vi "CDMA_RxDemodulate.vi"(8 "error in (no error)":errorcluster caption="错误输入（无错误）", 9 "pichData":cdb[](array[numeric]), 10 "dpchData":cdb[](array[numeric]), 11 "Path In":path) -> (0 "error out":errorcluster caption="错误输出", 1 "data1A":cdb[](array[numeric]), 2 "dpchBit":dbl[](array[numeric]), 3 "Path  Out":path)   [LabVIEW 2015]
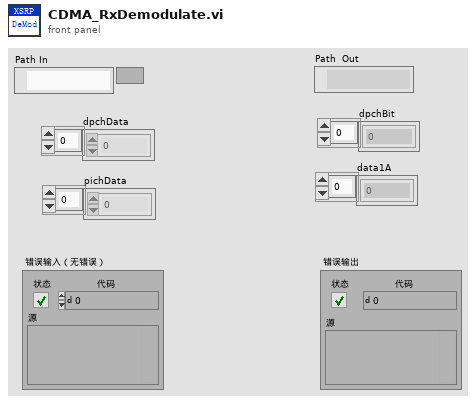
[diagram p1: front panel]
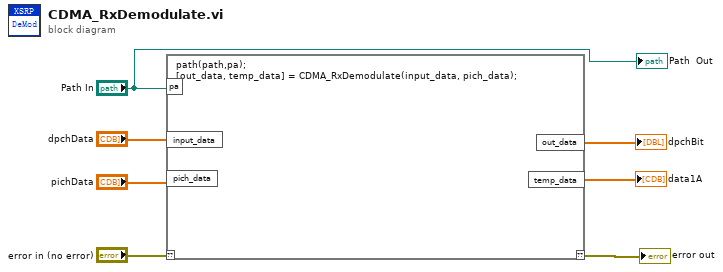
[diagram p0: block diagram]
diagram:
  n1 = script code="path(path,pa);\n[out_data, temp_data] = CDMA_RxDemodulate(input_data, pich_data);"("??"="error in (no error)", "pa"="Path In", "input_data"="dpchData", "pich_data"="pichData") -> ("??"=→"error out":errorcluster, "out_data"=→"dpchBit":dbl[], "temp_data"=→"data1A":cdb[])
  "Path  Out" <- "Path In"
